vi "Prototype.vi"() -> ()   [LabVIEW 2020]
uses:
  Newport Model 8742/New Focus Model 8742.lvclass
  SR 830 & NI USB7855R/SR 830 & NI USB7855R.lvclass
panel:
  out "Phase":dbl
  out "Amplitude":dbl
  in  "Acceleration (step/sec^2)":i32
  in  "Velocity (step/sec)":i32
  out "Current position (step)":i32
  in  "stop":bool
  out "is moving?":bool
  in  "Destination (steps)":i32=1000
  out "error out":errorcluster
  in  "error in":errorcluster
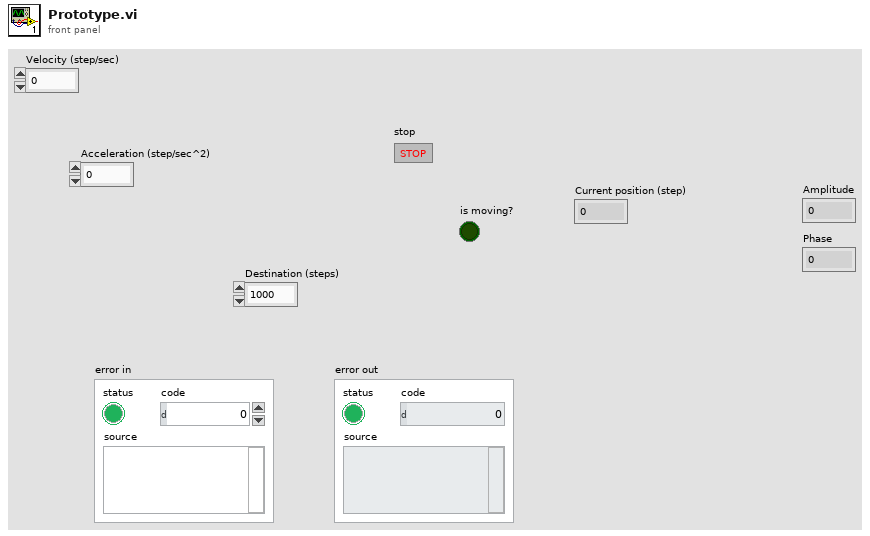
[diagram p1: front panel]
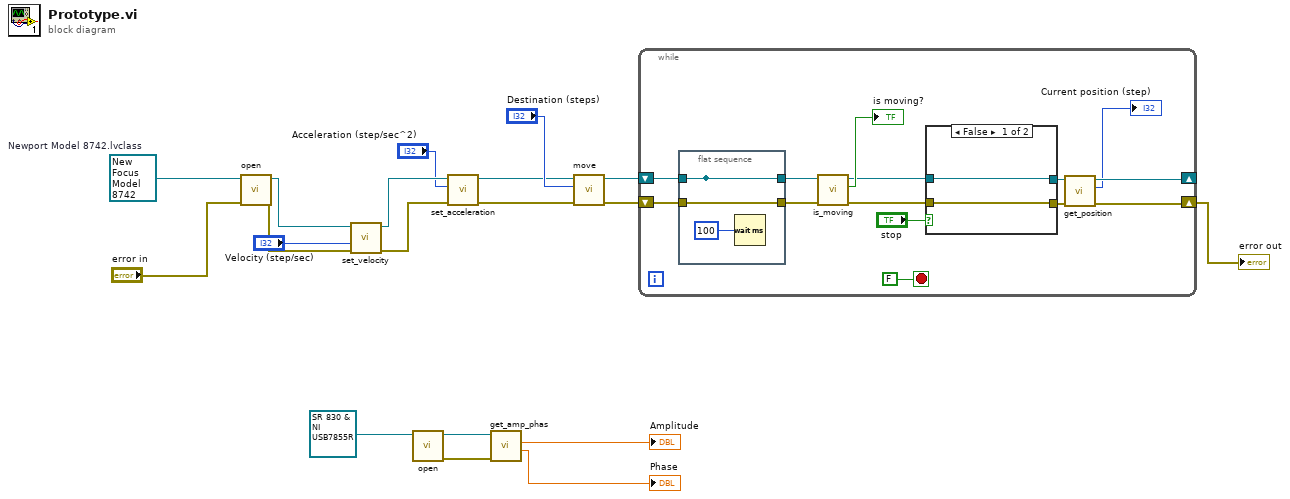
[diagram p0: block diagram]
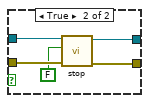
[diagram p2: hidden frame]
diagram:
  w19 = refnum<class "New Focus Model 8742.lvclass"> refnum  # Newport Model 8742.lvclass
  n1 = call-dynamic "open.vi"("error in (no error)"="error in", "Picomotor in"=w19) -> ("error out"=w12:errorcluster, "Picomotor out"=w13:refnum<class "New Focus Model 8742.lvclass">)  [unwired: 8 in]
  n2 = call-dynamic "set_velocity.vi"("error in (no error)"=w12, "Velocity (step/sec)"="Velocity (step/sec)", "Newport Model 8742 in"=w13) -> ("error out"=w8:errorcluster, "Newport Model 8742 out"=w7:refnum<class "New Focus Model 8742.lvclass">)  [unwired: 7 in]
  n3 = call-dynamic "open.vi"("Instrument in"=refnum<class "SR 830 & NI USB7855R.lvclass"> refnum ("SR 830 & NI USB7855R.lvclass")) -> ("error out"=w3:errorcluster, "Instrument out"=w4:refnum<class "SR 830 & NI USB7855R.lvclass">)  [unwired: 9 in]
  n4 = call-dynamic "set_acceleration.vi"("error in (no error)"=w8, "Acceleration (step/sec^2)"="Acceleration (step/sec^2)", "Newport Model 8742 in"=w7) -> ("error out"=w9:errorcluster, "Newport Model 8742 out"=w10:refnum<class "New Focus Model 8742.lvclass">)  [unwired: 7 in]
  n5 = call-dynamic "get_amp_phas.vi"("error in (no error)"=w3, "SR 830 & NI USB7855R in"=w4) -> ("Phase (rad)"=→"Phase":dbl, "Amplitude (V rms)"=→"Amplitude":dbl)  [unwired: 6 in, 2 out]
  n6 = call-dynamic "move.vi"("error in"=w9, "Destination (steps)"="Destination (steps)", "Newport Model 8742 in"=w10) -> ("error out"=w15:errorcluster, "Newport Model 8742 out"=w16:refnum<class "New Focus Model 8742.lvclass">)  [unwired: 7 in]
  n7 = while {
    shift-right: [w21] -> _
    shift-left: w16 -> [w32]
    shift-right: [w22] -> w14
    shift-left: w15 -> [w33]
    stop <- FALSE stop-if-true
    n8 = flat-sequence {
      tunnel: w33 -> [w42]
      tunnel: w32 -> [w41]
      tunnel: [w41] -> _
      tunnel: [w42] -> w30
      tunnel: [w41] -> w31
      frame #0 {
        n9 = Wait (ms)(milliseconds to wait=100) -> ()  [unwired: 1 out]
      }
    }
    n10 = call-dynamic "is_moving.vi"("error in"=w30, "Newport Model 8742 in"=w31) -> ("error out"=w26:errorcluster, "Is moving?"=→"is moving?":bool, "Newport Model 8742 out"=w27:refnum<class "New Focus Model 8742.lvclass">)  [unwired: 7 in]
    n11 = case shown="False" "stop" {
      tunnel: w27 -> [w35 w40]
      tunnel: w26 -> [w34 w39]
      tunnel: [w35 w38] -> w24
      tunnel: [w34 w37] -> w23
      frame False {
      }
      frame True {
        n12 = call "stop.vi"("error in (no error)"=w39, "Stop abruptly? (T)"=FALSE, "Picomotor in"=w40) -> ("error out"=w37:errorcluster, "Picomotor out"=w38:refnum<class "New Focus Model 8742.lvclass">)  [unwired: 7 in]
      }
    }
    n13 = call-dynamic "get_position.vi"("error in (no error)"=w23, "Newport Model 8742 in"=w24) -> ("error out"=w22:errorcluster, "Position (steps)"=→"Current position (step)":i32, "Newport Model 8742 out"=w21:refnum<class "New Focus Model 8742.lvclass">)  [unwired: 7 in]
  }
  "error out" <- w14
